vi "FFT1D(LabVIEW).vi"() -> ()   [LabVIEW 2020]
uses:
  ec656ee5-c5d1-4756-bc0c-4372cb75bedf.vi
  <vilib>/Analysis/2dsp.llb/Complex FFT.vi
  88f9a4a6-1eb4-4671-a21a-3a41d51d2300.vi
  <vilib>/Analysis/baseanly.llb/Mean (DBL).vi
  <vilib>/Utility/High Resolution Relative Seconds.vi
  <vilib>/Utility/file.llb/Write Delimited Spreadsheet (string).vi
  <vilib>/Analysis/NI_AALBase.lvlib
  <vilib>/Analysis/NI_AALPro.lvlib
panel:
  out "Results":dbl[](graph)=[0.008531578810346363, 0.018594736741904757, 0.04057894770276586, 0.09439999963720573, 0.2613210549737376, 0.6300999995896985, 1.2463578957402588, 2.628205262896556, 5.902831579748492, 17.379273683457683, 42.76611052658776, 92.63421052616506, 192.95122631516088, 423.0914500003564, 906.0349999999744, 2290.494699998817, 4152.274050000415, 7599.384250002913]
  in  "Benchmark Config":cluster{"Samples":i32, "Iteration":i32}[](array[cluster])=[{"Samples"=1024, "Iteration"=20}, {"Samples"=2048, "Iteration"=20}, {"Samples"=4096, "Iteration"=20}, {"Samples"=8192, "Iteration"=20}, {"Samples"=16384, "Iteration"=20}, {"Samples"=32768, "Iteration"=20}, {"Samples"=65536, "Iteration"=20}, {"Samples"=131072, "Iteration"=20}, {"Samples"=262144, "Iteration"=20}, {"Samples"=524288, "Iteration"=20}, {"Samples"=1048576, "Iteration"=20}, {"Samples"=2097152, "Iteration"=20}, {"Samples"=4194304, "Iteration"=20}, {"Samples"=8388608, "Iteration"=3}, {"Samples"=16777216, "Iteration"=3}, {"Samples"=33554432, "Iteration"=3}, {"Samples"=67108864, "Iteration"=3}, {"Samples"=134217728, "Iteration"=3}] {"Samples" format="%#.3p"}
  out "Results(s)":dbl[](array[numeric])=[0.008531578810346363, 0.018594736741904757, 0.04057894770276586, 0.09439999963720573, 0.2613210549737376, 0.6300999995896985, 1.2463578957402588, 2.628205262896556, 5.902831579748492, 17.379273683457683, 42.76611052658776, 92.63421052616506, 192.95122631516088, 423.0914500003564, 906.0349999999744, 2290.494699998817, 4152.274050000415, 7599.384250002913] format="%.8f"
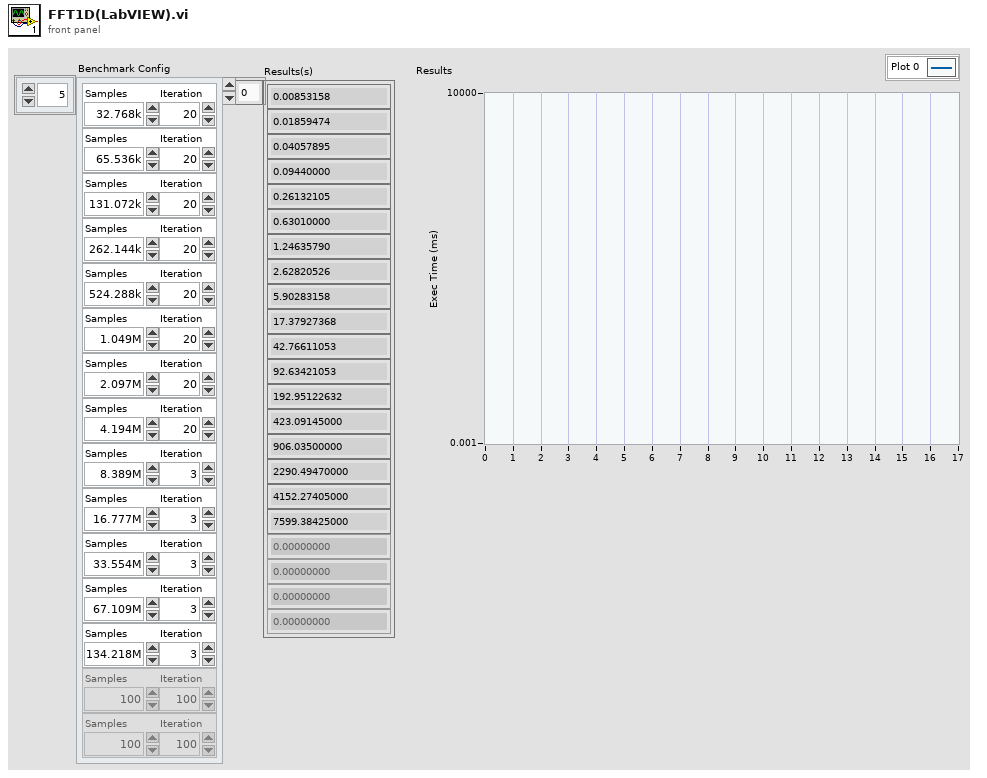
[diagram p1: front panel]
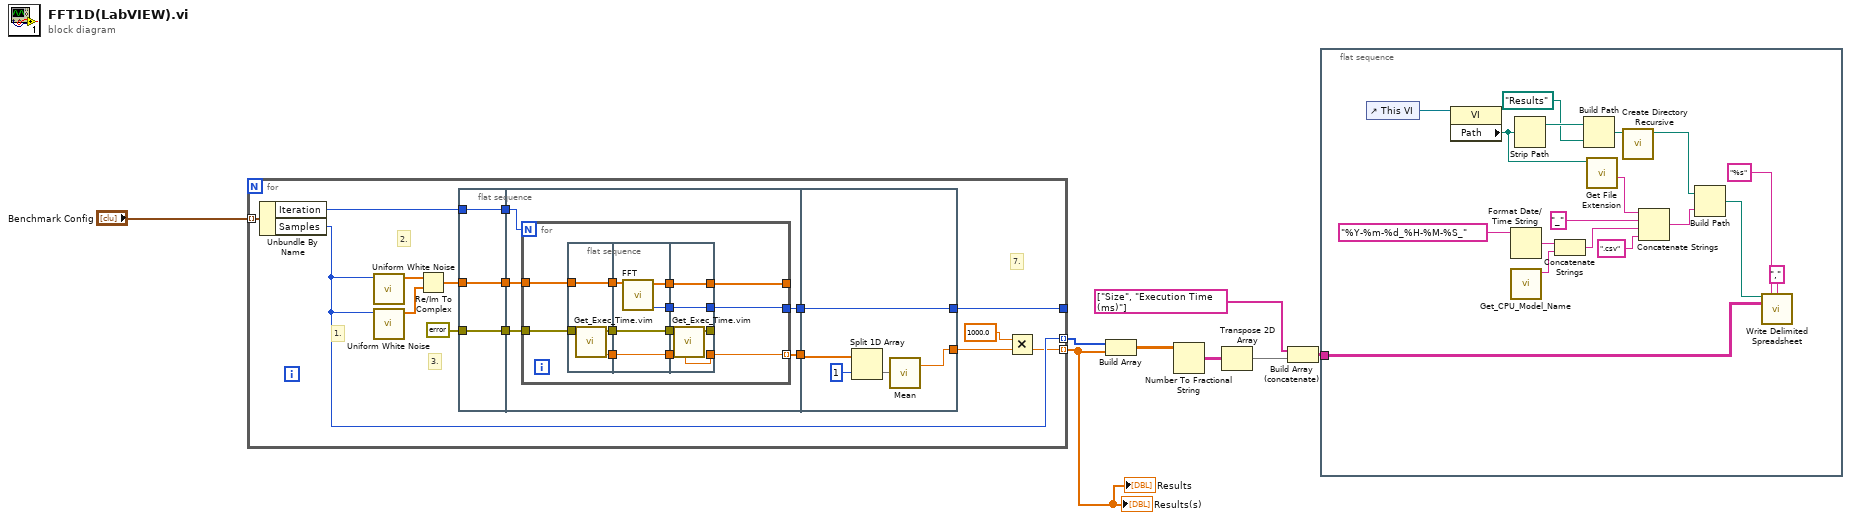
[diagram p0: block diagram]
diagram:
  n1 = for {
    tunnel: "Benchmark Config" -> [w24] mode=indexing
    tunnel: [w23] -> _
    tunnel: [w11] -> w1 mode=indexing
    tunnel: [w12] -> w3 mode=indexing
    # "3."
    # "7."
    # "2."
    # "1."
    n2 = Unbundle By Name(w24) -> ("Iteration"=w13:i32, "Samples"=w12:i32)
    n3 = call <vilib>:"Uniform White Noise.vi"("samples"=w12) -> ("uniform white noise"=w14:dbl[])  [unwired: 9 in, 1 out]
    n4 = call <vilib>:"Uniform White Noise.vi"("samples"=w12) -> ("uniform white noise"=w15:dbl[])  [unwired: 9 in, 1 out]
    n5 = Re/Im To Complex(1:w15, 2:w14) -> (0:w17:cdb[])
    n6 = flat-sequence {
      tunnel: errorcluster {"status"=FALSE, "code"=0, "source"=""} ("error out") -> [w25]
      tunnel: w17 -> [w26]
      tunnel: w13 -> [w27]
      tunnel: [w27] -> w21
      tunnel: [w26] -> w20
      tunnel: [w25] -> w19
      tunnel: [w30] -> w22
      tunnel: w21 -> [w29]
      tunnel: w20 -> [w32]
      tunnel: w19 -> [w31]
      tunnel: [w28] -> w9
      tunnel: [w64] -> w23
      tunnel: w22 -> [w64]
      tunnel: [w60] -> w18
      tunnel: w9 -> [w63]
      frame #0 {
      }
      frame #1 {
        n7 = for {
          N: w29 -> [_]
          tunnel: w32 -> [w43]
          tunnel: w31 -> [w41]
          tunnel: [w44] -> w30
          tunnel: [w42] -> _
          tunnel: [w33] -> w28 mode=indexing
          n8 = flat-sequence {
            tunnel: w41 -> [w47]
            tunnel: w43 -> [w48]
            tunnel: [w48] -> w40
            tunnel: [w46] -> w39
            tunnel: [w45] -> w34
            tunnel: w40 -> [w52]
            tunnel: w39 -> [w50]
            tunnel: [w53] -> w38
            tunnel: [w51] -> w37
            tunnel: [w50] -> w36
            tunnel: [w49] -> w35
            tunnel: w34 -> [w49]
            tunnel: [w56] -> _
            tunnel: [w58] -> w42
            tunnel: [w59] -> w44
            tunnel: w38 -> [w59]
            tunnel: w37 -> [w58]
            tunnel: w36 -> [w57]
            tunnel: w35 -> [w55]
            tunnel: [w54] -> w33
            frame #0 {
              n9 = call "Get_Exec_Time.vim"("error in (no error)"=w47) -> ("T(n)"=w45:dbl, "error out"=w46:errorcluster)  [unwired: 6 in, 1 out]
            }
            frame #1 {
              n10 = call-poly <vilib>:"FFT.vi"("X"=w52) -> ("error"=w53:i32, "FFT {X}"=w51:cdb[])  [unwired: 9 in]
            }
            frame #2 {
              n11 = call "Get_Exec_Time.vim"("T(n-1)"=w55, "error in (no error)"=w57) -> ("error out"=w56:errorcluster, "dT"=w54:dbl)  [unwired: 5 in, 1 out]
            }
          }
        }
      }
      frame #2 {
        n12 = Split 1D Array(array=w63, index=1) -> (second subarray=w61:dbl[])  [unwired: 1 out]
        n13 = call-poly <vilib>:"Mean.vi"("X"=w61) -> ("mean"=w60:dbl)  [unwired: 1 out]
      }
    }
    n14 = Multiply(x=1000.0, y=w18) -> (x*y=w11:dbl)
  }
  "Results(s)" <- w1
  "Results" <- w1
  n15 = Build Array(w3, w1) -> (w8:dbl[][])
  n16 = Number To Fractional String(number=w8) -> (F-format string=w7:string[][])  [unwired: 3 in]
  n17 = Transpose 2D Array(2D array=w7) -> (transposed array=w6:string[][])
  n18 = Build Array (concatenate)(string[] ["Size", "Execution Time (ms)"] ("element"), w6) -> (w2:string[][])
  n19 = flat-sequence {
    tunnel: w2 -> [w82]
    frame #0 {
      n20 = control-ref of="This VI"() -> (w76:refnum<vi>)
      n21 = property class="VI"(reference=w76) -> ("Path"=w71:path)  [unwired: 1 in, 2 out]
      n22 = Format Date/Time String(time format string (%c)="%Y-%m-%d_%H-%M-%S_") -> (date/time string=w67:string)  [unwired: 2 in]
      n23 = call "Get_CPU_Model_Name.vi"() -> ("CPU Model"=w66:string)  [unwired: 11 in]
      n24 = Strip Path(path=w71) -> (stripped path=w75:path)  [unwired: 1 out]
      n25 = Concatenate Strings(w67, w66) -> (w65:string)
      n26 = Build Path(base path=w75, name or relative path=path "Results") -> (appended path=w74:path)
      n27 = call <vilib>:"Get File Extension.vi"("file"=w71) -> ("filename without extension"=w70:string)  [unwired: 6 in, 4 out]
      n28 = call <vilib>:"Create Directory Recursive.vi"("directory"=w74) -> ("directory copy"=w72:path)  [unwired: 4 in, 2 out]
      n29 = Concatenate Strings(w70, "_" ("string"), w65, ".csv" ("string")) -> (w80:string)
      n30 = Build Path(base path=w72, name or relative path=w80) -> (appended path=w81:path)
      n31 = call-poly <vilib>:"Write Delimited Spreadsheet.vi"("file path (dialog if empty)"=w81, "format (%s)"="%s", "2D data"=w82, "delimiter (\\t)"="," ("delimiter (\\t)")) -> ()  [unwired: 10 in, 2 out]
    }
  }
